vi "Get Club Activities.vi"(8 "error in (no error)":errorcluster, 11 "Strava in":refnum<class "Strava curl.lvclass">) -> (0 "error out":errorcluster, 2 "Response":string, 3 "Strava out":refnum<class "Strava curl.lvclass">)   [LabVIEW 2020, in "Strava curl.lvclass"]
uses:
  Strava curl.lvclass
  Strava curl.lvclass/Strava curl.ctl
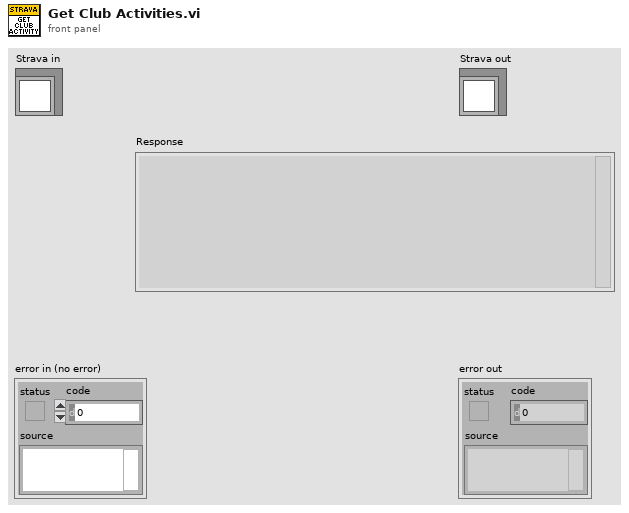
[diagram p1: front panel]
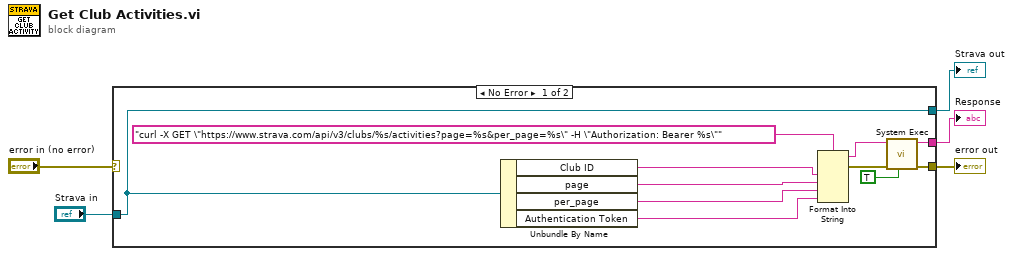
[diagram p0: block diagram]
diagram:
  n1 = case shown="No Error" "error in (no error)" {
    selector: "error in (no error)" -> [_ w18]
    tunnel: [w6 w18] -> w4
    tunnel: [w12 w17] -> w2
    tunnel: "Strava in" -> [w12 w17]
    tunnel: [w7 _] -> w1
    frame No Error {
      n2 = Unbundle By Name(w12) -> ("Club ID"=w11:string, "page"=w10:string, "per_page"=w9:string, "Authentication Token"=w8:string)
      n3 = Format Into String(format string="curl -X GET \"https://www.strava.com/api/v3/clubs/%s/activities?page=%s&per_page=%s\" -H \"Authorization: Bearer %s\"" ("command line"), w11, w10, w9, w8) -> (resulting string=w16:string, error out=w15:errorcluster)  [unwired: 2 in]
      n4 = call <vilib>:"System Exec.vi"("run minimized? (F)"=TRUE, "error in (no error)"=w15, "command line"=w16) -> ("error out"=w6:errorcluster, "standard output"=w7:string)  [unwired: 5 in, 2 out]
    }
    frame Error {
    }
  }
  "error out" <- w4
  "Strava out" <- w2
  "Response" <- w1
